vi "R11_22.vi"(9 "output valid in":bool, 10 "new_P11":fxp<+,32,16>, 11 "var_x":fxp<+,16,4>=1.0) -> (2 "output valid out":bool, 3 "R11":fxp<+,32,16>)   [LabVIEW 2020]
uses:
  <vilib>/rvi/FXPMathLib/FxpAdd/XNode/nifxpmath_Add.xnode
  <vilib>/rvi/FXPMathLib/sim/FxpSim.dll
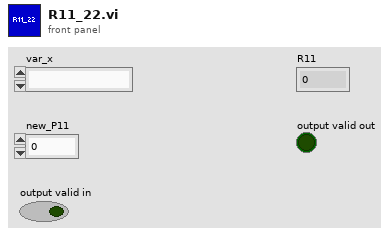
[diagram p1: front panel]
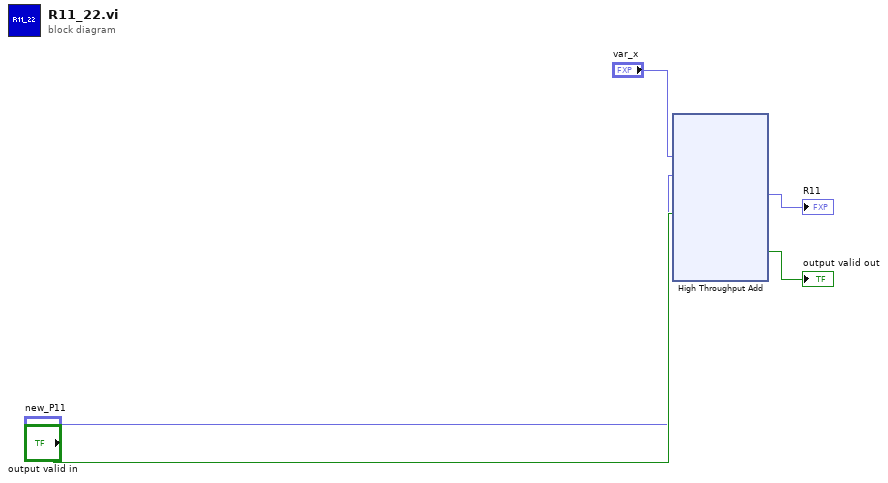
[diagram p0: block diagram]
diagram:
  n1 = xnode "High Throughput Add"("x"="var_x", "y"="new_P11", "input valid"="output valid in") -> ("x+y"=→"R11":fxp<+,32,16>, "output valid"=→"output valid out":bool)  [unwired: 1 in, 1 out]
